vi "Set Port Simulated.vi"(11 "Command to Send":string="SRC012;") -> (2 "output array":bool[](array[boolean]), 3 "Puerto":string)   [LabVIEW 2020, in "UI Actor.lvlib" / "UI Actor.lvclass"]
uses:
  UI Actor.lvclass
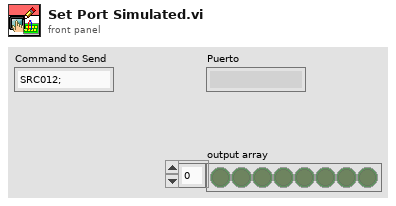
[diagram p1: front panel]
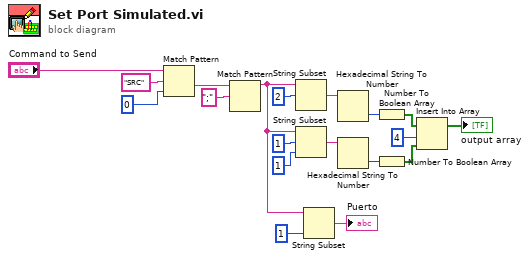
[diagram p0: block diagram]
diagram:
  n1 = Match Pattern(string="Command to Send", regular expression="SRC" ("string"), offset (0)=0) -> (after substring=w4:string)  [unwired: 3 out]
  n2 = Match Pattern(string=w4, regular expression=";") -> (before substring=w17:string)  [unwired: 1 in, 3 out]
  n3 = String Subset(string=w17, offset (0)=2) -> (substring=w10:string)  [unwired: 1 in]
  n4 = String Subset(string=w17, offset (0)=1, length (rest)=1 ("length (rest)")) -> (substring=w11:string)
  n5 = String Subset(string=w17, length (rest)=1 ("length (rest)")) -> (substring=→"Puerto":string)  [unwired: 1 in]
  n6 = Hexadecimal String To Number(string=w10) -> (number=w12:u32)  [unwired: 2 in, 1 out]
  n7 = Hexadecimal String To Number(string=w11) -> (number=w13:u32)  [unwired: 2 in, 1 out]
  n8 = Number To Boolean Array(number=w12) -> (Boolean array=w16:bool[])
  n9 = Number To Boolean Array(number=w13) -> (Boolean array=w15:bool[])
  n10 = Insert Into Array(array=w16, index=4, new element=w15) -> (→"output array":bool[])
